vi "Configure_Stations_Home.vi"() -> ()   [LabVIEW 2010]
uses:
  Motion_Gantry Position.ctl
  Motion_Coils Typedef.ctl
panel:
  out "error out":errorcluster
  in  "Gantry Move Data":T1={"Gantry Accel/Decel"=5.0, "Gantry Velocity"=5.0, "X-Position"=0.0, "Y-Position"=0.0, "Z-Position"=0.0} {"Z-Position" format="%_7g"; "Y-Position" format="%_7g"; "X-Position" format="%_7g"; "Gantry Velocity" format="%_7g"; "Gantry Accel/Decel" format="%_7g"}
  in  "TCP address:port (192.168.0.3:502)":string="192.168.0.3:502"
  in  "error in (no error)":errorcluster
  in  "Station Selection":T2(ring)=enum."Station 6 : Edwin"
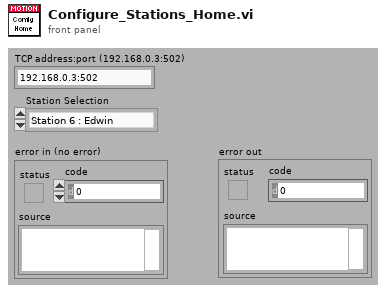
[diagram p1: front panel]
types:
  T1 = typedef "Motion_Gantry Position.ctl" = cluster{"Gantry Accel/Decel":dbl, "Gantry Velocity":dbl, "X-Position":dbl, "Y-Position":dbl, "Z-Position":dbl}
  T2 = enum16{"Station 2 : Benjamin", "Station 6 : Edwin"}
  T3 = typedef "Motion_Coils Typedef.ctl" = u16
  T4 = cluster{"Approach Velocity\n(In/Sec)":dbl, "Creep Velocity\n(In/Sec)":dbl, "Offset (In)":dbl, "OffsetVelocity\n(In/Sec)":dbl, "AccDec\n(In/Sec/Sec)":dbl, "Position (In)":dbl}
  T5 = cluster{"Approach Velocity (In/Sec)":dbl, "Creep Velocity (In/Sec)":dbl, "Offset (In)":dbl, "OffsetVelocity (In/Sec)":dbl, "AccDec\n(In/Sec/Sec)":dbl, "Position (In)":dbl}
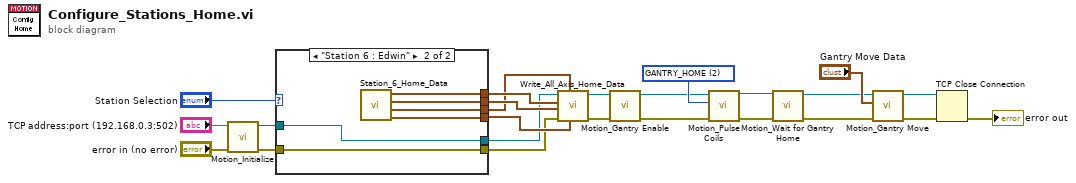
[diagram p0: block diagram]
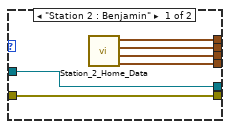
[diagram p2: hidden frame]
diagram:
  w19 = T3 2 items=["GANTRY_ALARM_CLEAR", "GANTRY_ENABLE", "GANTRY_HOME", "GANTRY_GOTO", "LOADER_HOME", "LOADER_ALARM_CLEAR", "LOADER_ENABLE", "LOADER_GOTO_CONNECT", "LOADER_GOTO_LOAD", "LOADER_STOP"] ("Coils")
  n1 = call "Motion_Initialize.vi"("error in (no error)"="error in (no error)", "TCP address:port (192.168.0.3:502)"="TCP address:port (192.168.0.3:502)") -> ("error out"=w18:errorcluster, "connection ID"=w16:refnum<k5>)  [unwired: 8 in]
  n2 = case shown="\"Station 6 : Edwin\"" "Station Selection" {
    tunnel: [w30 w36] -> w23
    tunnel: [w29 w35] -> w22
    tunnel: [w28 w34] -> w20
    tunnel: [w27 w33] -> w21
    tunnel: [w25 w32] -> w17
    tunnel: w18 -> [w25 w32]
    tunnel: [w26 w31] -> w15
    tunnel: w16 -> [w26 w31]
    frame "Station 2 : Benjamin" {
      n3 = call "Station_2_Home_Data.vi"() -> ("Loader Home Data OUT"=w27:T4, "Z Home Data OUT"=w28:T4, "Y Home Data OUT"=w29:T4, "X Home Data OUT"=w30:T5)  [unwired: 8 in]
    }
    frame "Station 6 : Edwin" {
      n4 = call "Station_6_Home_Data.vi"() -> ("Loader Home Data OUT"=w33:T4, "Z Home Data OUT"=w34:T4, "Y Home Data OUT"=w35:T4, "X Home Data OUT"=w36:T5)  [unwired: 8 in]
    }
  }
  n5 = call "Write_All_Axis_Home_Data.vi"("Loader Home Data"=w21, "Z Home Data"=w20, "error in (no error)"=w17, "Y Home Data"=w22, "X Home Data"=w23, "TCP Connection Refnum in"=w15) -> ("error out"=w9:errorcluster, "TCP Connection Refnum out"=w7:refnum<k5>)  [unwired: 4 in]
  n6 = call "Motion_Gantry Enable.vi"("error in (no error)"=w9, "TCP Connection Refnum in"=w7) -> ("error out"=w8:errorcluster, "TCP Connection Refnum (dup)"=w6:refnum<k5>)  [unwired: 8 in]
  n7 = call "Motion_Pulse Coils.vi"("error in"=w8, "Pulse Coil"=w19, "TCP refnum"=w6) -> ("error out"=w2:errorcluster, "TCP refnum dup"=w4:refnum<k5>)  [unwired: 7 in]
  n8 = call "Motion_Wait for Gantry Home.vi"("error in"=w2, "TCP refnum"=w4) -> ("error out"=w1:errorcluster, "TCP refnum dup"=w3:refnum<k5>)  [unwired: 4 in, 4 out]
  n9 = call "Motion_Gantry Move.vi"("error in (no error)"=w1, "Gantry Move Data"="Gantry Move Data", "TCP Connection Refnum in"=w3) -> ("error out"=w12:errorcluster, "TCP Connection Refnum (dup)"=w11:refnum<k5>)  [unwired: 7 in]
  n10 = TCP Close Connection(connection ID=w11, error in (no error)=w12) -> (error out=→"error out":errorcluster)  [unwired: 1 in, 1 out]
